vi "Rayleigh CDF.vi"(10 "b":dbl=1.0, 11 "x":dbl=1.0) -> (0 "error":i32, 3 "cdf(x)":dbl=0.3934693402873666)   [LabVIEW 2018, in "NI_Gmath.lvlib"]
doc: "Computes the continuous cumulative distribution function (CDF), or the probability that the random variate X, where X describes the selected distribution type, has a value less than or equal to <B>x</B>. You must manually select the polymorphic instance to use."
uses:
  NI_Gmath.lvlib
  st_error_code.ctl
panel:
  # "Rayleigh CDF"
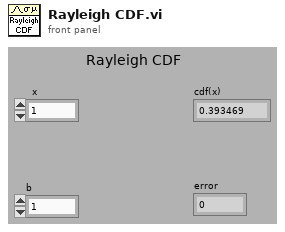
[diagram p1: front panel]
types:
  T1 = typedef "NI_Gmath.lvlib/st_error_code.ctl" = i32
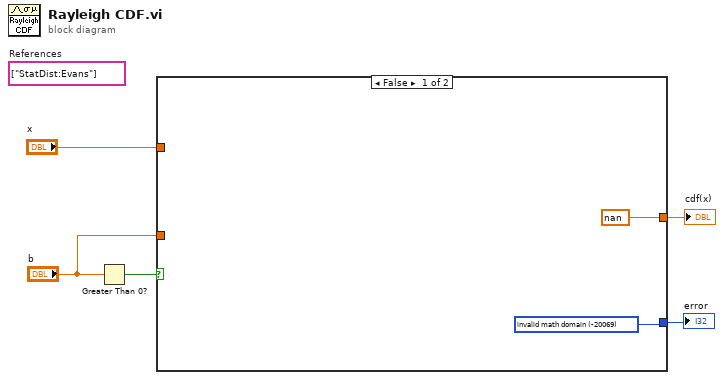
[diagram p0: block diagram]
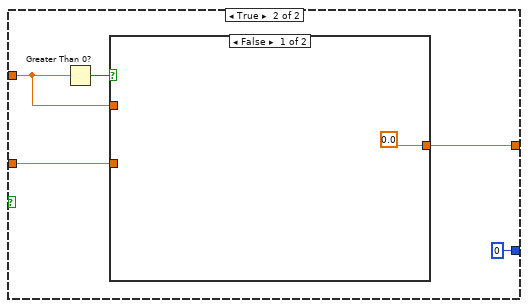
[diagram p2: hidden frame]
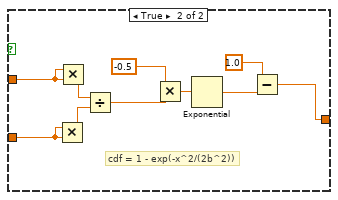
[diagram p3: hidden frame]
diagram:
  (unwired) string[] ["StatDist:Evans"]  # References
  n1 = Greater Than 0?(x="b") -> (x > 0?=w2:bool)
  n2 = case shown="False" w2 {
    tunnel: "b" -> [_ w10]
    tunnel: [w6 0 ("invalid math domain")] -> w5
    tunnel: [nan w11] -> w4
    tunnel: "x" -> [_ w8]
    frame False {
      w6 = T1 -20069 items=["invalid math domain"=-20069, "Fourier interpolation size m >= n"=-20070, "empty array"=-20003] ("stat interp error code")
    }
    frame True {
      n3 = Greater Than 0?(x=w8) -> (x > 0?=w9:bool)
      n4 = case shown="False" w9 {
        tunnel: [0.0 w21] -> w11
        tunnel: w8 -> [_ w20]
        tunnel: w10 -> [_ w17]
        frame False {
        }
        frame True {
          # "cdf = 1 - exp(-x^2/(2b^2))"
          n5 = Multiply(x=w17, y=w17) -> (x*y=w18:dbl)
          n6 = Multiply(x=w20, y=w20) -> (x*y=w19:dbl)
          n7 = Divide(x=w19, y=w18) -> (x/y=w15:dbl)
          n8 = Multiply(x=-0.5, y=w15) -> (x*y=w14:dbl)
          n9 = Exponential(1:w14) -> (0:w23:dbl)
          n10 = Subtract(x=1.0, y=w23) -> (x-y=w21:dbl)
        }
      }
    }
  }
  "cdf(x)" <- w4
  "error" <- w5
